vi "Keithley2400series_MUX_2_Set Ch.vi"(2 "Err In":errorcluster, 3 "On/Off":bool, 4 "Channal":u8 max=7, 5 "VISA In":refnum<visa-resource-name>) -> (0 "Err Out":errorcluster, 1 "VISA Out":refnum<visa-resource-name>)   [LabVIEW 2014]
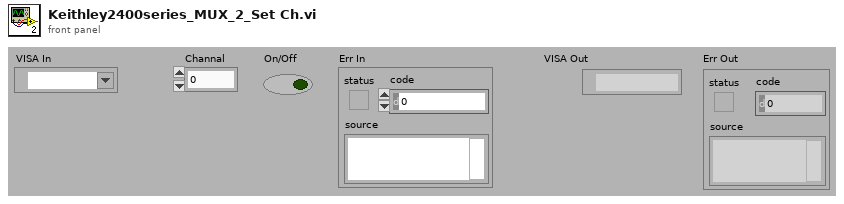
[diagram p1: front panel]
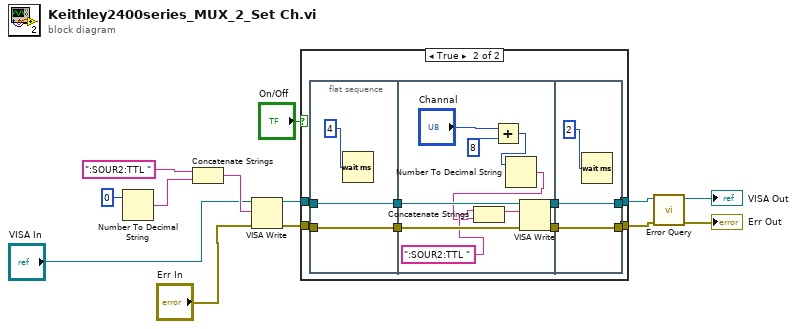
[diagram p0: block diagram]
diagram:
  n1 = Number To Decimal String(number=0) -> (decimal integer string=w8:string)  [unwired: 1 in]
  n2 = Concatenate Strings(":SOUR2:TTL " ("string"), w8) -> (w6:string)
  n3 = VISA Write(VISA resource name="VISA In", write buffer=w6, error in (no error)="Err In") -> (VISA resource name out=w11:refnum<visa-resource-name>, error out=w13:errorcluster)  [unwired: 1 out]
  n4 = case shown="True" "On/Off" {
    tunnel: [w15 w23] -> w10
    tunnel: w11 -> [w15 w21]
    tunnel: [w14 w22] -> w12
    tunnel: w13 -> [w14 w20]
    frame False {
    }
    frame True {
      n5 = flat-sequence {
        tunnel: w20 -> [w25]
        tunnel: w21 -> [w26]
        tunnel: [w26] -> w19
        tunnel: [w25] -> w18
        tunnel: w19 -> [w32]
        tunnel: w18 -> [w31]
        tunnel: [w34] -> w17
        tunnel: [w33] -> w16
        tunnel: [w38] -> w22
        tunnel: [w39] -> w23
        tunnel: w17 -> [w39]
        tunnel: w16 -> [w38]
        frame #0 {
          n6 = Wait (ms)(milliseconds to wait=u32 4) -> ()  [unwired: 1 out]
        }
        frame #1 {
          n7 = Add(x="Channal", y=u8 8) -> (x+y=w28:u8)
          n8 = Number To Decimal String(number=w28) -> (decimal integer string=w27:string)  [unwired: 1 in]
          n9 = Concatenate Strings(":SOUR2:TTL " ("string"), w27) -> (w30:string)
          n10 = VISA Write(VISA resource name=w32, write buffer=w30, error in (no error)=w31) -> (VISA resource name out=w34:refnum<visa-resource-name>, error out=w33:errorcluster)  [unwired: 1 out]
        }
        frame #2 {
          n11 = Wait (ms)(milliseconds to wait=u32 2) -> ()  [unwired: 1 out]
        }
      }
    }
  }
  n12 = call "Error Query.vi"("error in (no error)"=w12, "VISA resource name"=w10) -> ("error out"=→"Err Out":errorcluster, "VISA resource name out"=→"VISA Out":refnum<visa-resource-name>)  [unwired: 6 in, 2 out]
